vi "PPSU Values.vi"(8 "error in":errorcluster, 11 "PPSU Queue":refnum<queue>) -> (0 "Fehler":errorcluster caption="Error out")   [LabVIEW 2022 SP3]
uses:
  6D_Global.vi
panel:
  out "Read data 3":string
  out "Read data (hex) 2":u8[](array[numeric]) format="%.0x"
  out "Read data 2":string
  out "Read data (hex)":u8[](array[numeric]) format="%.0x"
  out "Read data":string
  out "array 2":string[](array[string])
  out "match substring":string
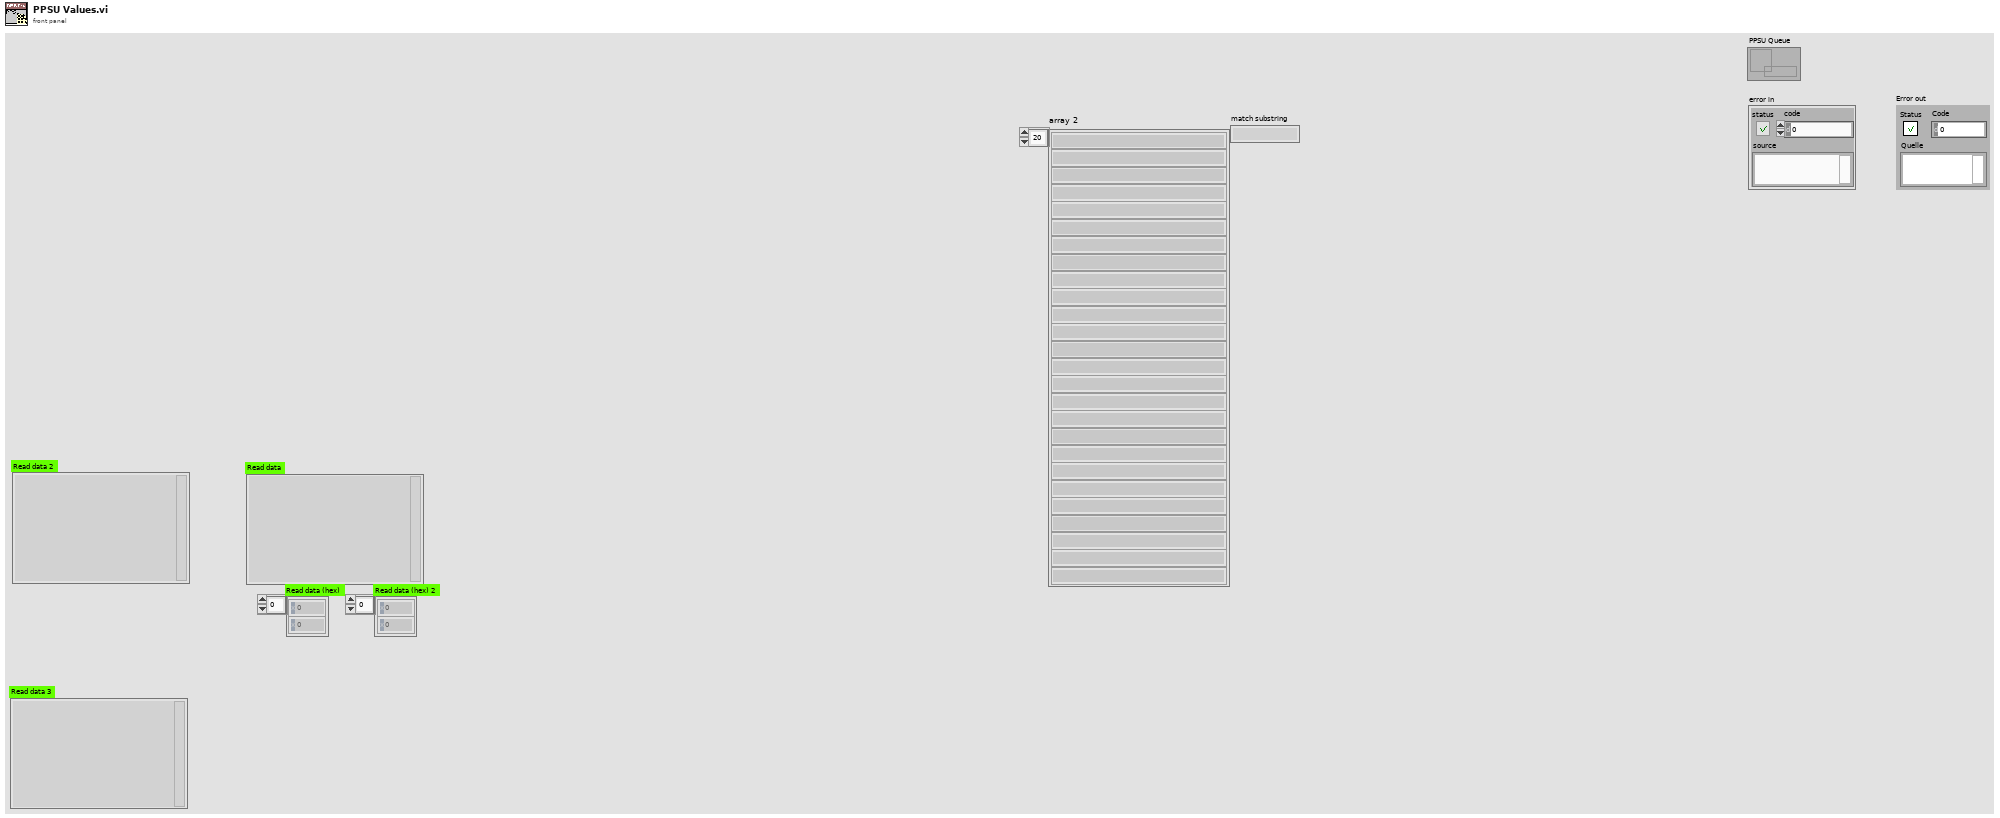
[diagram p1: front panel]
types:
  T1 = cluster{"Alarm":bool, "Power Fail":bool, "OVD":bool, "OCD":bool, "OPD":bool, "MSP":bool}
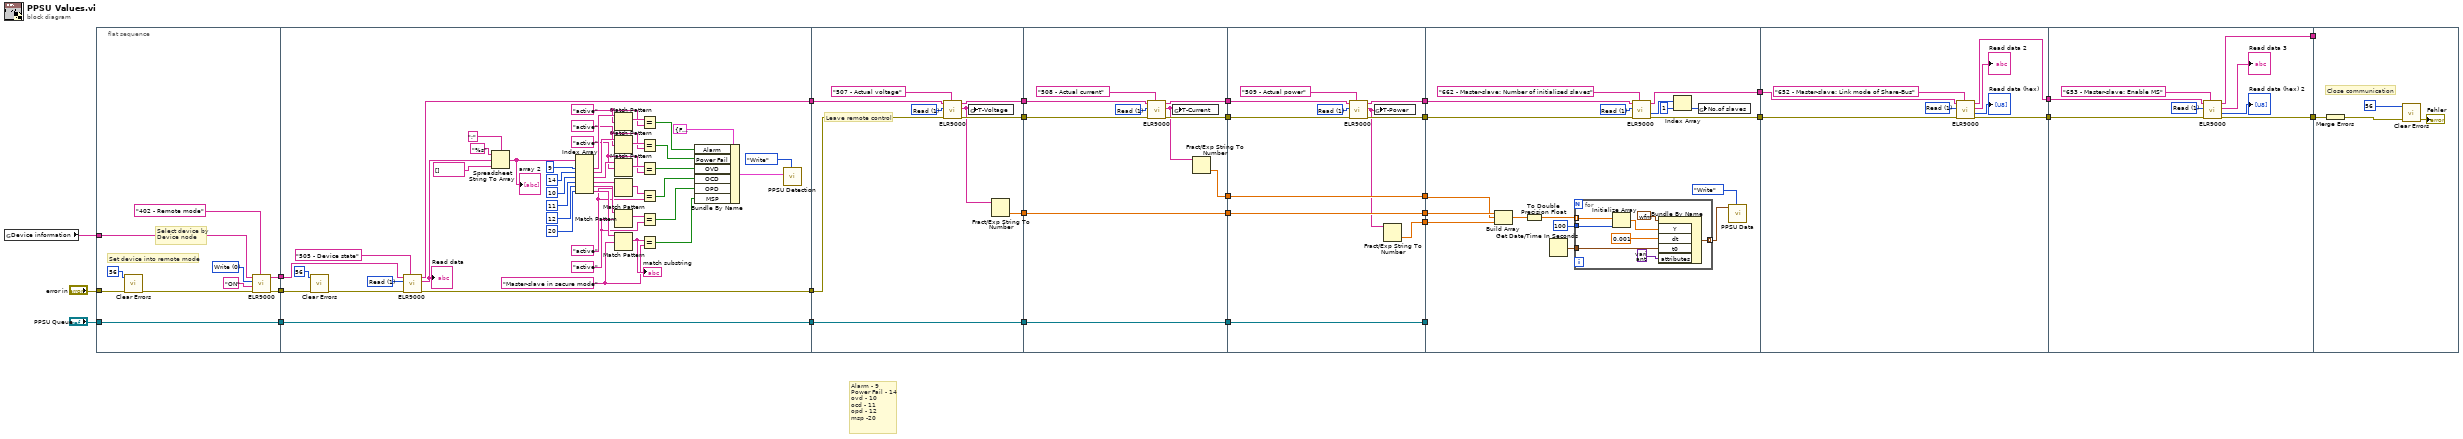
[diagram p0: block diagram]
diagram:
  # "Alarm - 9\nPower Fail - 14\novd - 10\nocd - 11\nopd - 12\nmsp -20"
  n1 = global read "6D_Global.vi" "Device information"() -> (w13:string[])
  n2 = flat-sequence {
    tunnel: [w40] -> w29
    tunnel: [w39] -> w30
    tunnel: w13 -> [w35]
    tunnel: "error in" -> [w33]
    tunnel: "PPSU Queue" -> [w31]
    tunnel: [w31] -> w5
    tunnel: [w87] -> w28
    tunnel: w30 -> [w84]
    tunnel: w29 -> [w83]
    tunnel: [w52] -> w27
    tunnel: w5 -> [w41]
    tunnel: [w41] -> w4
    tunnel: [w92] -> w26
    tunnel: w28 -> [w94]
    tunnel: [w93] -> w25
    tunnel: w27 -> [w91]
    tunnel: [w88] -> w12
    tunnel: w4 -> [w90]
    tunnel: [w90] -> w3
    tunnel: w26 -> [w102]
    tunnel: [w101] -> w24
    tunnel: w25 -> [w103]
    tunnel: [w104] -> w23
    tunnel: w12 -> [w100]
    tunnel: [w100] -> w11
    tunnel: [w97] -> w10
    tunnel: w3 -> [w99]
    tunnel: [w99] -> w2
    tunnel: w24 -> [w113]
    tunnel: [w112] -> w22
    tunnel: w23 -> [w115]
    tunnel: [w114] -> w21
    tunnel: w11 -> [w110]
    tunnel: w10 -> [w111]
    tunnel: [w107] -> w9
    tunnel: [w111] -> w8
    tunnel: [w110] -> w7
    tunnel: w2 -> [w109]
    tunnel: [w109] -> w1
    tunnel: w22 -> [w133]
    tunnel: [w132] -> w20
    tunnel: w21 -> [w134]
    tunnel: [w135] -> w19
    tunnel: w9 -> [w124]
    tunnel: w8 -> [w125]
    tunnel: w7 -> [w126]
    tunnel: w1 -> [_]
    tunnel: w20 -> [w149]
    tunnel: [w148] -> w18
    tunnel: w19 -> [w151]
    tunnel: [w150] -> w17
    tunnel: w18 -> [w157]
    tunnel: [w156] -> w16
    tunnel: w17 -> [w159]
    tunnel: [w158] -> w15
    tunnel: w16 -> [w163]
    tunnel: w15 -> [_]
    frame #0 {
      w38 = u8 0 items=["Write", "Read"] ("Access")
      # "Select device by\nDevice node"
      # "Set device into remote mode"
      n3 = call <vilib>:"Clear Errors.vi"("error in (no error)"=w33, "specific error code to clear (0: all)"=56) -> ("error out"=w34:errorcluster)  [unwired: 4 in, 1 out]
      n4 = call <vilib>:"ELR9000.vi"("Command list"="402 - Remote mode", "Error in"=w34, "Value"="ON", "Access"=w38, "Device information in"=w35) -> ("Error out"=w40:errorcluster, "Device information out"=w39:string[])  [unwired: 1 in, 2 out]
    }
    frame #1 {
      w64 = "Master-slave in secure mode" ("regular expression")
      w51 = "active" ("regular expression")
      w63 = "active" ("regular expression")
      w62 = "active" ("regular expression")
      w61 = "active" ("regular expression")
      w60 = "active" ("regular expression")
      w86 = u8 1 items=["Write", "Read"] ("Access")
      n5 = call <vilib>:"Clear Errors.vi"("error in (no error)"=w83, "specific error code to clear (0: all)"=56) -> ("error out"=w78:errorcluster)  [unwired: 4 in, 1 out]
      n6 = call <vilib>:"ELR9000.vi"("Command list"="505 - Device state", "Error in"=w78, "Access"=w86, "Device information in"=w84) -> ("Error out"=w52:errorcluster, "Read data"=w82:string, "Device information out"=w87:string[])  [unwired: 2 in, 1 out]
      "Read data" <- w82
      n7 = Spreadsheet String To Array(delimiter (Tab)=";", format string="%s", spreadsheet string=w82, array type (2D Dbl)=string[] []) -> (array=w53:string[])
      "array 2" <- w53
      n8 = Index Array(array=w53, index #1=9 ("index"), index #2=14 ("index"), index #3=10 ("index"), index #4=11 ("index"), index #5=12 ("index"), index #6=20 ("index")) -> (element #1=w71:string, element #2=w72:string, element #3=w73:string, element #4=w74:string, element #5=w75:string, element #6=w76:string)
      n9 = Match Pattern(string=w71, regular expression=w60) -> (match substring=w65:string)  [unwired: 1 in, 3 out]
      n10 = Match Pattern(string=w72, regular expression=w61) -> (match substring=w66:string)  [unwired: 1 in, 3 out]
      n11 = Match Pattern(string=w73, regular expression=w62) -> (match substring=w67:string)  [unwired: 1 in, 3 out]
      n12 = Match Pattern(string=w74, regular expression=w51) -> (match substring=w69:string)  [unwired: 1 in, 3 out]
      n13 = Match Pattern(string=w75, regular expression=w63) -> (match substring=w68:string)  [unwired: 1 in, 3 out]
      n14 = Match Pattern(string=w76, regular expression=w64) -> (match substring=w70:string)  [unwired: 1 in, 3 out]
      "match substring" <- w70
      n15 = Equal?(x=w65, y=w60) -> (x = y?=w47:bool)
      n16 = Equal?(x=w66, y=w61) -> (x = y?=w46:bool)
      n17 = Equal?(x=w67, y=w62) -> (x = y?=w45:bool)
      n18 = Equal?(x=w69, y=w51) -> (x = y?=w44:bool)
      n19 = Equal?(x=w68, y=w63) -> (x = y?=w43:bool)
      n20 = Equal?(x=w70, y=w64) -> (x = y?=w42:bool)
      n21 = Bundle By Name(cluster=T1 {"Alarm"=FALSE, "Power Fail"=FALSE, "OVD"=FALSE, "OCD"=FALSE, "OPD"=FALSE, "MSP"=FALSE} ("PPSU Dect"), "Alarm"=w47, "Power Fail"=w46, "OVD"=w45, "OCD"=w44, "OPD"=w43, "MSP"=w42) -> (w48:T1)
      n22 = call "PPSU Detection.vi"("Write/Read"=enum16{"Write", "Read"}."Write", "PPSU Dect"=w48) -> ()  [unwired: 8 in, 2 out]
    }
    frame #2 {
      w96 = u8 1 items=["Write", "Read"] ("Access")
      # "Leave remote control"
      n23 = call <vilib>:"ELR9000.vi"("Command list"="507 - Actual voltage", "Error in"=w91, "Access"=w96, "Device information in"=w94) -> ("Error out"=w92:errorcluster, "Read data"=w89:string, "Device information out"=w93:string[])  [unwired: 2 in, 1 out]
      n24 = global write "6D_Global.vi" "T-Voltage"(w89) -> ()
      n25 = Fract/Exp String To Number(string=w89) -> (number=w88:dbl)  [unwired: 3 in, 1 out]
    }
    frame #3 {
      w105 = u8 1 items=["Write", "Read"] ("Access")
      n26 = call <vilib>:"ELR9000.vi"("Command list"="508 - Actual current", "Error in"=w102, "Access"=w105, "Device information in"=w103) -> ("Error out"=w101:errorcluster, "Read data"=w98:string, "Device information out"=w104:string[])  [unwired: 2 in, 1 out]
      n27 = global write "6D_Global.vi" "T-Current"(w98) -> ()
      n28 = Fract/Exp String To Number(string=w98) -> (number=w97:dbl)  [unwired: 3 in, 1 out]
    }
    frame #4 {
      w117 = u8 1 items=["Write", "Read"] ("Access")
      n29 = call <vilib>:"ELR9000.vi"("Command list"="509 - Actual power", "Error in"=w113, "Access"=w117, "Device information in"=w115) -> ("Error out"=w112:errorcluster, "Read data"=w108:string, "Device information out"=w114:string[])  [unwired: 2 in, 1 out]
      n30 = global write "6D_Global.vi" "T-Power"(w108) -> ()
      n31 = Fract/Exp String To Number(string=w108) -> (number=w107:dbl)  [unwired: 3 in, 1 out]
    }
    frame #5 {
      w130 = u8 1 items=["Write", "Read"] ("Access")
      n32 = Build Array(w126, w125, w124) -> (w123:dbl[])
      n33 = To Double Precision Float(number=w123) -> (double precision float=w120:dbl[])
      n34 = Get Date/Time In Seconds() -> (seconds since 1Jan1904=w122:timestamp)
      n35 = for {
        tunnel: w120 -> [w143] mode=indexing
        tunnel: 100 ("dimension size") -> [w142]
        tunnel: [w138] -> w118 mode=indexing
        tunnel: w122 -> [w136]
        n36 = Initialize Array(w143, w142) -> (w141:dbl[])
        n37 = Bundle By Name(cluster=waveform(dbl) {"t0"=timestamp(0 s since 1904-01-01), "dt"=1.0, "Y"=[]} ("waveform"), "Y"=w141, "dt"=0.001, "t0"=w136, "attributes"=variant) -> (w138:waveform(dbl))
      }
      n38 = call <vilib>:"ELR9000.vi"("Command list"="662 - Master-slave: Number of initialised slaves", "Error in"=w133, "Access"=w130, "Device information in"=w134) -> ("Error out"=w132:errorcluster, "Read data (hex)"=w129:u8[], "Device information out"=w135:string[])  [unwired: 2 in, 1 out]
      n39 = Index Array(array=w129, index=1) -> (element=w127:u8)
      n40 = global write "6D_Global.vi" "No.of slaves"(w127) -> ()
      n41 = call "PPSU Data.vi"("Write/Read"=enum16{"Write", "Read"}."Write", "PPSU Data"=w118) -> ()  [unwired: 9 in, 1 out]
    }
    frame #6 {
      w147 = u8 1 items=["Write", "Read"] ("Access")
      n42 = call <vilib>:"ELR9000.vi"("Command list"="652 - Master-slave: Link mode of Share-Bus", "Error in"=w149, "Access"=w147, "Device information in"=w151) -> ("Error out"=w148:errorcluster, "Read data (hex)"=→"Read data (hex)":u8[], "Read data"=→"Read data 2":string, "Device information out"=w150:string[])  [unwired: 2 in]
    }
    frame #7 {
      w155 = u8 1 items=["Write", "Read"] ("Access")
      n43 = call <vilib>:"ELR9000.vi"("Command list"="653 - Master-slave: Enable MS", "Error in"=w157, "Access"=w155, "Device information in"=w159) -> ("Error out"=w156:errorcluster, "Read data (hex)"=→"Read data (hex) 2":u8[], "Read data"=→"Read data 3":string, "Device information out"=w158:string[])  [unwired: 2 in]
    }
    frame #8 {
      # "Close communication"
      n44 = Merge Errors(w163) -> (w160:errorcluster)
      n45 = call <vilib>:"Clear Errors.vi"("error in (no error)"=w160, "specific error code to clear (0: all)"=56) -> ("error out"=→"Fehler":errorcluster)  [unwired: 4 in, 1 out]
    }
  }
